vi "Filter new data.vi"(6 "Tree and Table":refnum<vi>, 7 "Headers":string[](array[string]), 8 "error in":errorcluster, 10 "Data IN":string[][](array[string]), 11 "Filter":refnum<vi>) -> (0 "error out":errorcluster, 3 "Filtered Array":string[][](array[string]))   [LabVIEW 2025]
uses:
  <vilib>/Utility/error.llb/whitespace.ctl
  <vilib>/Utility/error.llb/Trim Whitespace One-Sided.vi
  Table_Filtering/Table_Filtering.lvlib
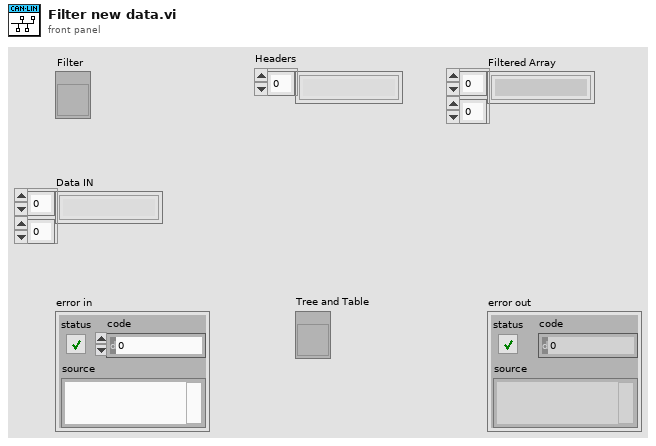
[diagram p1: front panel]
types:
  T1 = typedef "whitespace.ctl" = u16
  T2 = cluster{"FIELD":string, "OPERATOR":string, "VALUE":string}[]
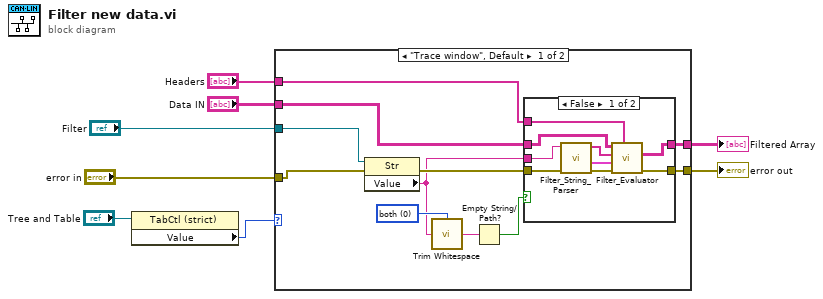
[diagram p0: block diagram]
diagram:
  n1 = property class="TabCtl (strict)"(reference="Tree and Table") -> ("Value"=w3:enum32{"Trace window", "Signal table"})  [unwired: 1 in, 2 out]
  n2 = case shown="\"Trace window\", Default" w3 {
    tunnel: [w18 w31] -> w8
    tunnel: [w15 w32] -> w7
    tunnel: "error in" -> [w12 w31]
    tunnel: "Filter" -> [w11 _]
    tunnel: "Headers" -> [w10 _]
    tunnel: "Data IN" -> [w9 w32]
    frame "Trace window", Default {
      w16 = T1 0 items=["both", "start of string", "end of string"] ("location (both)")
      n3 = property class="Str"(reference=w11, error in=w12) -> (error out=w19:errorcluster, "Value"=w13:string)  [unwired: 1 out]
      n4 = call <vilib>:"Trim Whitespace.vi"("string"=w13, "location (both)"=w16) -> ("trimmed string"=w17:string)
      n5 = Empty String/Path?(string/path=w17) -> (empty?=w14:bool)
      n6 = case shown="False" w14 {
        tunnel: w19 -> [w28 w29]
        tunnel: [w27 w29] -> w18
        tunnel: w9 -> [w25 w30]
        tunnel: [w22 w30] -> w15
        tunnel: w13 -> [w21 _]
        tunnel: w10 -> [w20 _]
        frame False {
          n7 = call "Filter_String_Parser.vi"("error in"=w28, "Filter String"=w21) -> ("error constant"=w26:errorcluster, "Comparators"=w23:T2, "Boolean Connectors"=w24:string[])  [unwired: 7 in]
          n8 = call "Filter_Evaluator.vi"("Headers"=w20, "Error"=w26, "Comparators"=w23, "Boolean Connectors"=w24, "Prefiltered Data"=w25) -> ("Error Out"=w27:errorcluster, "Filtered Array"=w22:string[][])  [unwired: 4 in, 1 out]
        }
        frame True {
        }
      }
    }
    frame "Signal table" {
    }
  }
  "error out" <- w8
  "Filtered Array" <- w7
